vi "test_libssh2_session_banner_get.vi"() -> ()   [LabVIEW 2017, in "integration_tests.lvlib"]
uses:
  integration_tests.lvlib
  support/support.lvlib
  libssh2/libssh2.lvlib
  <vilib>/PNR/Transparent Assertions/Transparent Assertions/Transparent Assertions.lvlib
panel:
  out "error out":errorcluster
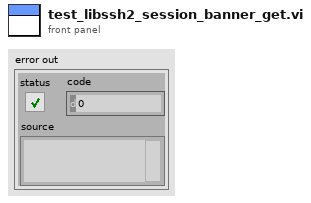
[diagram p1: front panel]
types:
  T1 = typedef "libssh2.lvlib/Session Refnum.ctl" = refnum<k1>
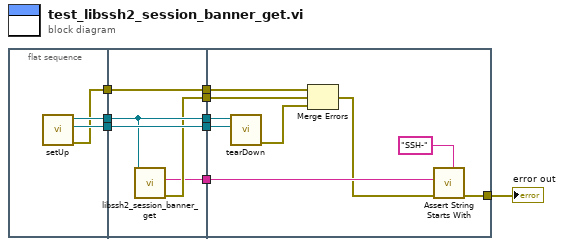
[diagram p0: block diagram]
diagram:
  n1 = flat-sequence {
    tunnel: [w12] -> w9
    tunnel: [w11] -> w8
    tunnel: [w10] -> w7
    tunnel: w9 -> [w15]
    tunnel: w8 -> [w17]
    tunnel: [w15] -> w6
    tunnel: [w17] -> w5
    tunnel: w7 -> [w16]
    tunnel: [w16] -> w4
    tunnel: [w14] -> w3
    tunnel: [w13] -> w2
    tunnel: w6 -> [w26]
    tunnel: w5 -> [w25]
    tunnel: w4 -> [w23]
    tunnel: w3 -> [w22]
    tunnel: w2 -> [w21]
    tunnel: [w19] -> w1
    frame #0 {
      n2 = call "setUp.vi"() -> ("error out"=w10:errorcluster, "connection ID"=w11:refnum<k5>, "session"=w12:T1)  [unwired: 9 in]
    }
    frame #1 {
      n3 = call "libssh2_session_banner_get.vi"("session"=w15) -> ("error out"=w14:errorcluster, "banner"=w13:string)  [unwired: 9 in]
    }
    frame #2 {
      n4 = call "tearDown.vi"("connection ID"=w25, "session"=w26) -> ("error out"=w24:errorcluster)  [unwired: 9 in]
      n5 = Merge Errors(w23, w22, w24) -> (w20:errorcluster)
      n6 = call <vilib>:"Assert String Starts With.vi"("Prefix"="SSH-", "error in (no error)"=w20, "String"=w21) -> ("error out"=w19:errorcluster)  [unwired: 8 in]
    }
  }
  "error out" <- w1
